vi "Initialise.vi"(8 "error in (no error)":errorcluster, 10 "frame":string="/world", 11 "MF3 in":refnum<class "MF3.lvclass">) -> (0 "error out":errorcluster, 3 "MF3 out":refnum<class "MF3.lvclass">)   [LabVIEW 2011, in "MF3.lvclass"]
uses:
  MF3.lvclass
  controls/Drive Status.ctl
  <vilib>/LabVIEW Targets/FPGA/cRIO/cRIO-9505/controls.llb/_nicrio_cRIO-9505_DriveStatus.ctl
  controls/5-bar Parameters.ctl
  MF3.lvclass/MF3.ctl
  <vilib>/FPGAPlugInAG/NI 9157/niLvFpga_Open_NI 9157.vi
  <vilib>/Utility/error.llb/Error Cluster From Error Code.vi
  <vilib>/rvi/errors/niLvFpgaAdjustHostInterfaceError.vi
  <vilib>/rvi/interface/nirviOpenFPGA/nirviOpenFPGA.xnode
  FPGA/MotorsInterface.lvbitx
  <vilib>/rvi/interface/nirviReadWriteControl/nirviReadWriteControl.xnode
  Finger/Finger.lvclass
  NiFpgaLv.dll
panel:
  out "Motors Status":T1[](array[typedef])=[{"Status"=enum."Enabled", "Vsup Present"=FALSE, "Drive Fault"=FALSE, "Temp Fault"=FALSE}, {"Status"=enum."Enabled", "Vsup Present"=FALSE, "Drive Fault"=FALSE, "Temp Fault"=FALSE}, {"Status"=enum."Enabled", "Vsup Present"=FALSE, "Drive Fault"=FALSE, "Temp Fault"=FALSE}, {"Status"=enum."Enabled", "Vsup Present"=FALSE, "Drive Fault"=FALSE, "Temp Fault"=FALSE}, {"Status"=enum."Enabled", "Vsup Present"=FALSE, "Drive Fault"=FALSE, "Temp Fault"=FALSE}, {"Status"=enum."Enabled", "Vsup Present"=FALSE, "Drive Fault"=FALSE, "Temp Fault"=FALSE}, {"Status"=enum."Enabled", "Vsup Present"=FALSE, "Drive Fault"=FALSE, "Temp Fault"=FALSE}, {"Status"=enum."Enabled", "Vsup Present"=FALSE, "Drive Fault"=FALSE, "Temp Fault"=FALSE}, {"Status"=enum."Enabled", "Vsup Present"=FALSE, "Drive Fault"=FALSE, "Temp Fault"=FALSE}, {"Status"=enum."Enabled", "Vsup Present"=FALSE, "Drive Fault"=FALSE, "Temp Fault"=FALSE}]
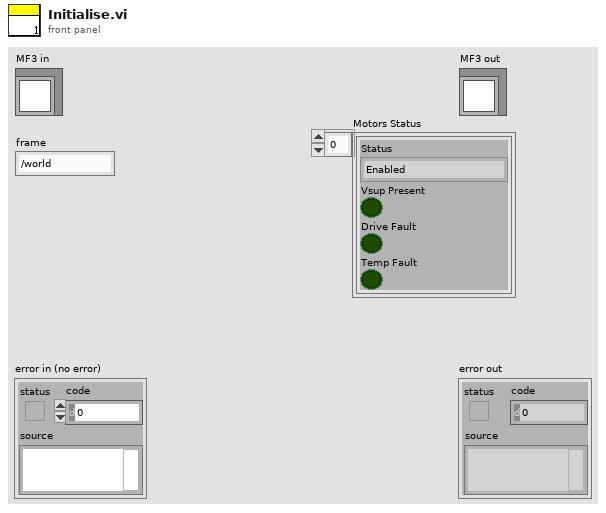
[diagram p1: front panel]
types:
  T1 = typedef "Drive Status.ctl" = cluster{"Status":T2, "Vsup Present":bool, "Drive Fault":bool, "Temp Fault":bool}
  T2 = typedef "_nicrio_cRIO-9505_DriveStatus.ctl" = enum8{"Enabled", "Disabled", "Disabled by Drive Fault", "Disabled by Temp. Fault", "Disabled by E-Stop", "Unknown"}
  T3 = typedef "5-bar Parameters.ctl" = cluster{"distances":cluster{"L1":dbl, "L2":dbl, "L3":dbl, "L4":dbl, "d":dbl, "d6":dbl}, "angles":cluster{"phi":dbl, "theta":dbl, "psi":dbl, "alpha":dbl}}
  T4 = cluster{"initial_angles":sgl[], "directions":sgl[]}
  T5 = typedef "Dynamic Parameters.ctl" = cluster{"gear_ratios":sgl[]}
  T6 = typedef "NI_Robotics_Link.lvclass/Joint Type.ctl" = enum16{"Revolute", "Prismatic"}
  T7 = typedef "5-bar Side.ctl" = enum16{"Left", "Right"}
  T8 = cluster{"Thumb":cluster{"k":sgl[][], "p":sgl[][], "T0":sgl[][], "types":T6[], "side":T7}, "Middle":cluster{"k":sgl[][], "p":sgl[][], "T0":sgl[][], "types":T6[], "side":T7}, "Index":cluster{"k":sgl[][], "p":sgl[][], "T0":sgl[][], "types":T6[], "side":T7}}
  T9 = cluster{"k":sgl[][], "p":sgl[][], "T0":sgl[][], "types":T6[], "side":T7}
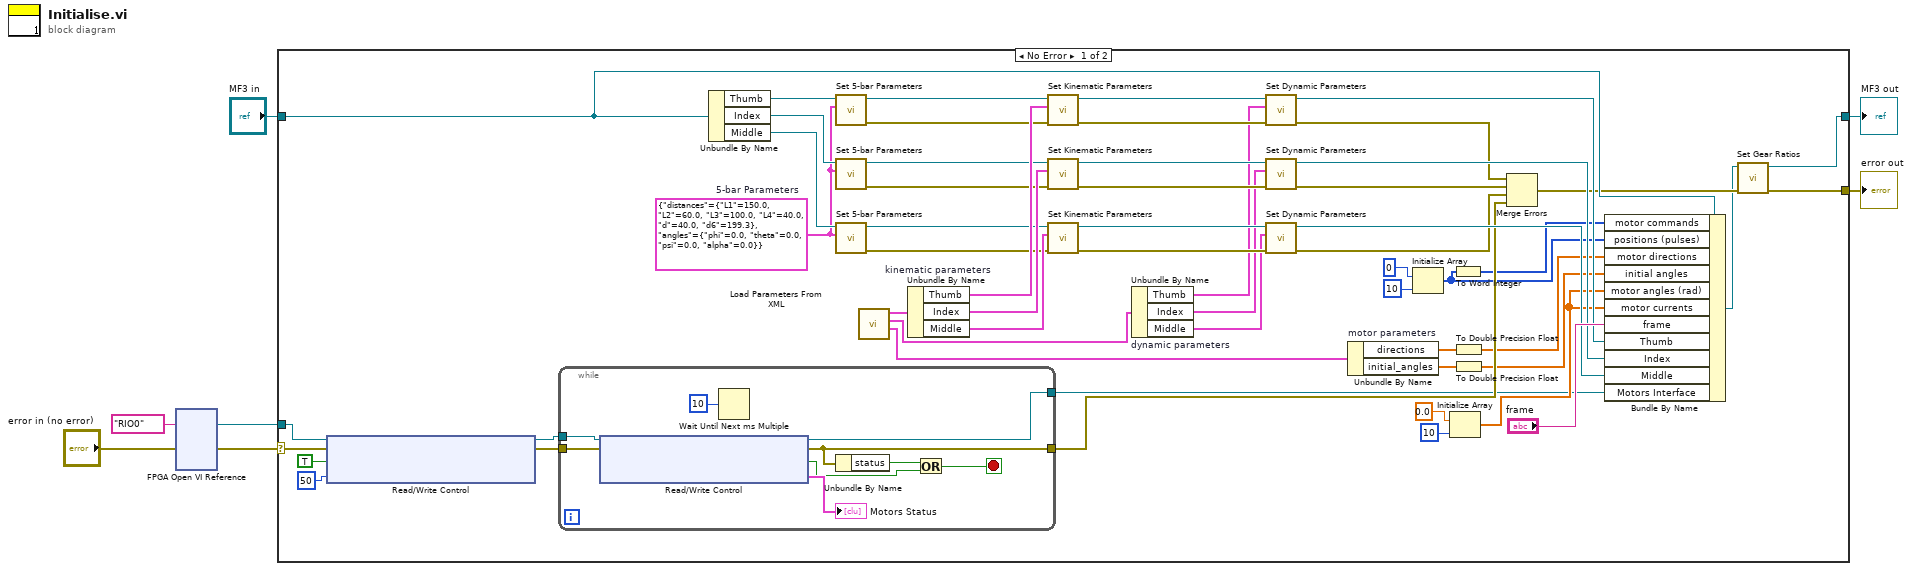
[diagram p0: block diagram]
diagram:
  n1 = xnode "FPGA Open VI Reference"("error in"="error in (no error)", "resource name"=tag "RIO0") -> ("FPGA VI Reference Out"=w2:refnum<k20>, "error out"=w3:errorcluster)
  n2 = case shown="No Error" w3 {
    selector: w3 -> [w58 w74]
    tunnel: [w18 w74] -> w7
    tunnel: [w17 w73] -> w5
    tunnel: "MF3 in" -> [w56 w73]
    tunnel: w2 -> [w63 _]
    frame No Error {
      w20 = T3 {"distances"={"L1"=150.0, "L2"=60.0, "L3"=100.0, "L4"=40.0, "d"=40.0, "d6"=199.3}, "angles"={"phi"=0.0, "theta"=0.0, "psi"=0.0, "alpha"=0.0}}  # 5-bar Parameters
      n3 = xnode "Read/Write Control"("FPGA VI Reference In"=w63, "error in"=w58, "Enable Motors"=TRUE, "Current Loop Rate (usec)"=u32 50) -> ("FPGA VI Reference Out"=w61:refnum<k20>, "error out"=w60:errorcluster)
      n4 = while {
        tunnel: w61 -> [w72]
        tunnel: w60 -> [w71]
        tunnel: [w70] -> w15
        tunnel: [w67] -> w36
        stop <- w65 stop-if-true
        n5 = xnode "Read/Write Control"("FPGA VI Reference In"=w72, "error in"=w71) -> ("FPGA VI Reference Out"=w70:refnum<k20>, "error out"=w67:errorcluster, "All Enabled"=w68:bool, "Motors Status"=→"Motors Status":T1[])
        n6 = Wait Until Next ms Multiple(millisecond multiple=u32 10) -> ()  [unwired: 1 out]
        n7 = Unbundle By Name(w67) -> ("status"=w66:bool)
        n8 = Or(x=w66, y=w68) -> (x .or. y?=w65:bool)
      }
      n9 = Unbundle By Name(w56) -> ("Thumb"=w22:refnum<class "Finger.lvclass">, "Index"=w21:refnum<class "Finger.lvclass">, "Middle"=w27:refnum<class "Finger.lvclass">)
      n10 = call "Set 5-bar Parameters.vi"("5-bar Parameters"=w20, "Finger in"=w22) -> ("error out"=w23:errorcluster, "Finger out"=w24:refnum<class "Finger.lvclass">)  [unwired: 8 in]
      n11 = call "Set 5-bar Parameters.vi"("5-bar Parameters"=w20, "Finger in"=w21) -> ("error out"=w25:errorcluster, "Finger out"=w26:refnum<class "Finger.lvclass">)  [unwired: 8 in]
      n12 = call "Set 5-bar Parameters.vi"("5-bar Parameters"=w20, "Finger in"=w27) -> ("error out"=w28:errorcluster, "Finger out"=w29:refnum<class "Finger.lvclass">)  [unwired: 8 in]
      n13 = call "Load Parameters From XML.vi"() -> ("motor parameters"=w12:T4, "dynamic parameters"=w44:cluster{"Thumb":T5, "Middle":T5, "Index":T5}, "kinematic parameters"=w40:T8)  [unwired: 8 in, 1 out]
      n14 = Unbundle By Name "kinematic parameters"(w40) -> ("Thumb"=w39:T9, "Index"=w38:T9, "Middle"=w37:T9)
      n15 = call "Set Kinematic Parameters.vi"("error in (no error)"=w23, "kinematic parameters"=w39, "Finger in"=w24) -> ("error out"=w54:errorcluster, "Finger out"=w53:refnum<class "Finger.lvclass">)  [unwired: 7 in]
      n16 = call "Set Kinematic Parameters.vi"("error in (no error)"=w25, "kinematic parameters"=w38, "Finger in"=w26) -> ("error out"=w51:errorcluster, "Finger out"=w45:refnum<class "Finger.lvclass">)  [unwired: 7 in]
      n17 = call "Set Kinematic Parameters.vi"("error in (no error)"=w28, "kinematic parameters"=w37, "Finger in"=w29) -> ("error out"=w49:errorcluster, "Finger out"=w50:refnum<class "Finger.lvclass">)  [unwired: 7 in]
      n18 = Unbundle By Name "dynamic parameters"(w44) -> ("Thumb"=w43:T5, "Index"=w41:T5, "Middle"=w42:T5)
      n19 = call "Set Dynamic Parameters.vi"("error in (no error)"=w54, "dynamic parameters"=w43, "Finger in"=w53) -> ("error out"=w33:errorcluster, "Finger out"=w55:refnum<class "Finger.lvclass">)  [unwired: 7 in]
      n20 = call "Set Dynamic Parameters.vi"("error in (no error)"=w51, "dynamic parameters"=w41, "Finger in"=w45) -> ("error out"=w34:errorcluster, "Finger out"=w52:refnum<class "Finger.lvclass">)  [unwired: 7 in]
      n21 = call "Set Dynamic Parameters.vi"("error in (no error)"=w49, "dynamic parameters"=w42, "Finger in"=w50) -> ("error out"=w35:errorcluster, "Finger out"=w48:refnum<class "Finger.lvclass">)  [unwired: 7 in]
      n22 = Unbundle By Name "motor parameters"(w12) -> ("directions"=w11:sgl[], "initial_angles"=w10:sgl[])
      n23 = Initialize Array(0 ("Position Thumb 1"), 10 ("dimension size")) -> (w14:i32[])
      n24 = Initialize Array(0.0 ("element"), 10 ("dimension size")) -> (w32:dbl[])
      n25 = To Word Integer(number=w14) -> (16bit integer=w13:i16[])
      n26 = To Double Precision Float(number=w11) -> (double precision float=w9:dbl[])
      n27 = To Double Precision Float(number=w10) -> (double precision float=w8:dbl[])
      n28 = Merge Errors(w33, w34, w35, w36) -> (w19:errorcluster)
      n29 = Bundle By Name(cluster=w56, "motor commands"=w13, "positions (pulses)"=w14, "motor directions"=w9, "initial angles"=w8, "motor angles (rad)"=w32, "motor currents"=w32, "frame"="frame", "Thumb"=w55, "Index"=w52, "Middle"=w48, "Motors Interface"=w15) -> (w16:refnum<class "MF3.lvclass">)
      n30 = call "Set Gear Ratios.vi"("error in (no error)"=w19, "MF3 in"=w16) -> ("error out"=w18:errorcluster, "MF3 out"=w17:refnum<class "MF3.lvclass">)  [unwired: 8 in]
    }
    frame Error {
    }
  }
  "error out" <- w7
  "MF3 out" <- w5
